vi "ConnectionDetails.vi"(8 "error in (no error)":errorcluster) -> (0 "error out":errorcluster, 3 "Connection Details":T1)   [LabVIEW 2019, in "MicronTemplateAPIs.lvlib" / "MicronTemplateAPIs.lvclass"]
uses:
  MicronTemplateAPIs.lvclass
  vi.lib/Micron/Base/Client/Typedefs/ServiceDetails.ctl
  vi.lib/Micron/Base/Client/MicronClient.lvclass
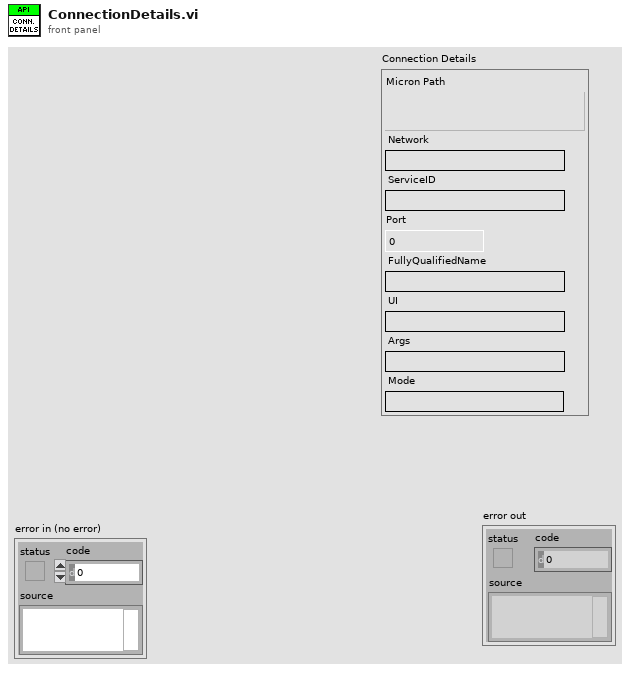
[diagram p1: front panel]
types:
  T1 = typedef "MicronClient.lvclass/ServiceDetails.ctl" = cluster{"Micron Path":path, "Network":string, "ServiceID":string, "Port":i32, "FullyQualifiedName":string, "UI":string, "Args":string, "Mode":string}
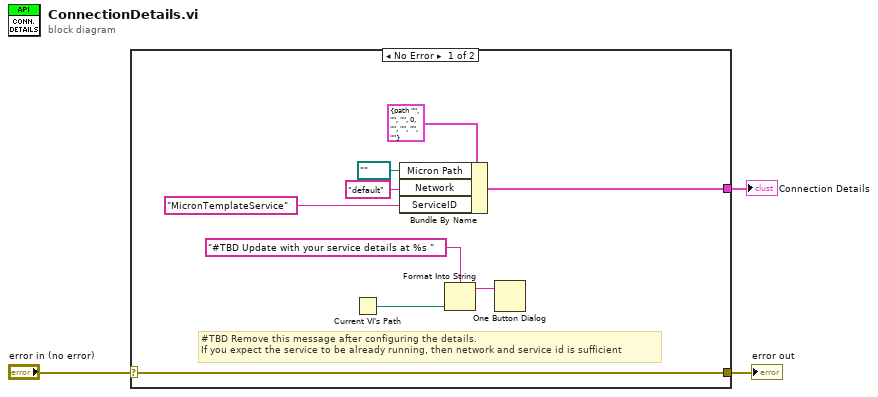
[diagram p0: block diagram]
diagram:
  n1 = case shown="No Error" "error in (no error)" {
    selector: "error in (no error)" -> [w12 w13]
    tunnel: [w12 w13] -> w2
    tunnel: [w10 _] -> w1
    frame No Error {
      # "#TBD Remove this message after configuring the details.\nIf you expect the service to be already running, then network and service id is sufficient"
      n2 = Current VI's Path() -> (path=w5:path)
      n3 = Bundle By Name(cluster=T1 {"Micron Path"=path "", "Network"="", "ServiceID"="", "Port"=0, "FullyQualifiedName"="", "UI"="", "Args"="", "Mode"=""} ("Connection Details"), "Micron Path"=path "", "Network"="default", "ServiceID"="MicronTemplateService") -> (w10:T1)
      n4 = Format Into String(format string="#TBD Update with your service details at %s " ("message"), w5) -> (resulting string=w4:string)  [unwired: 2 in, 1 out]
      n5 = One Button Dialog(message=w4) -> ()  [unwired: 1 in, 1 out]
    }
    frame Error {
    }
  }
  "error out" <- w2
  "Connection Details" <- w1
